vi "HitrapGUI.HTLE_TR6-UpperPart.vi"() -> ()   [LabVIEW 2014, in "HitrapGUI.lvlib"]
uses:
  HitrapGUI.lvlib
  CSlibraries/GUILib/GUILib.userEventsMainType.ctl
  CSlibraries-extern/DimLVEvent/DimIndicators/DimIndicators.anyType.ctl
  CSlibraries/GUILib/GUILib.simpleNumeric.ctl
  CSlibraries/GUILib/GUILib.basicNumeric.ctl
  CSlibraries-extern/DimLVEvent/DimIndicators/DimIndicators.numericType.ctl
  CSlibraries/UtilityLib/UtilityLib.valueStatus.ctl
  CS_Core/CSSystem/CoreDefs/CoreDefs.rawDataType.ctl
  CS_Core/CSSystem/CoreLib/CoreLib.int 2 byte array.vi
  CS_Core/CSSystem/CoreLib/CoreLib.double 2 byte array.vi
  CSlibraries/UtilityLib/UtilityLib.lvlib
  CS_Core/CSSystem/CSSystemLib/CSSystemLib.lvlib
  CSlibraries-extern/DimLVEvent/DimIndicators/DimIndicators.lvlib
  CS_Core/GUIs/GOGControllerGUI/GOGControllerGUI.lvlib
  CSlibraries/GUILib/GUILib.lvlib
  CS_Core/CSSystem/CoreLib/CoreLib.lvlib
  CSlibraries-extern/DimLVEvent/LVDimInterface/LVDimInterface.lvlib
panel:
  in  "MotorActivityLink-Act":T1
  in  "MotorLink-Act":T1
  in  "TR6DK4Link":T2
  in  "TR6DK5Link":T2
  in  "TR6ME1Ctl 2":T3 caption="TR6QME1" {"nom" step=1.0}
  in  "TR6ME1Ctl":T3 caption="TR6QME1" {"nom" step=1.0}
  in  "TR6QD4_1Ctl":T3 caption="TR6QD4_1" {"nom" step=1.0}
  in  "TR6QD4_2Ctl":T3 caption="TR6QD4_2" {"nom" step=1.0}
  in  "TR6KY5Ctl":T3 caption="TR6KY5" {"nom" step=1.0}
  in  "TR6KX5Ctl":T3 caption="TR6KX5" {"nom" step=1.0}
  in  "TR6KY4Ctl":T3 caption="TR6KY4" {"nom" step=1.0}
  in  "TR6KX4Ctl":T3 caption="TR6KX4" {"nom" step=1.0}
  in  "TR6DK5Ctl":T5 caption="TR6DK5" {"Progress Slide" scale=0.0..100.0; "Nom_Position" items=["Undefined", "Open", "Faraday Cup", "MCP"]}
  in  "TR6DK4Ctl":T5 caption="TR6DK4" {"Progress Slide" scale=0.0..100.0; "Nom_Position" items=["Undefined", "Open", "Faraday Cup", "MCP"]}
  in  "userEventsMain 2":T6
  in  "userEventsMain":T6
  in  "Next":bool
  in  "Previous":bool
  in  "analog1Ctl":T3 {"nom" step=1.0}
  in  "analog1":bool=TRUE
  out "subSystem1State":string
  in  "subSystem1":bool
  out "subSystem1StateQuality":string
  in  "subControllersIgnoredDIM":T1
  in  "iniData":string
  in  "stop":bool
  in  "dummy":bool
  in  "parentSystem":bool
  in  "userEvent":refnum<user-event>
  # "TR6-UpperPart"
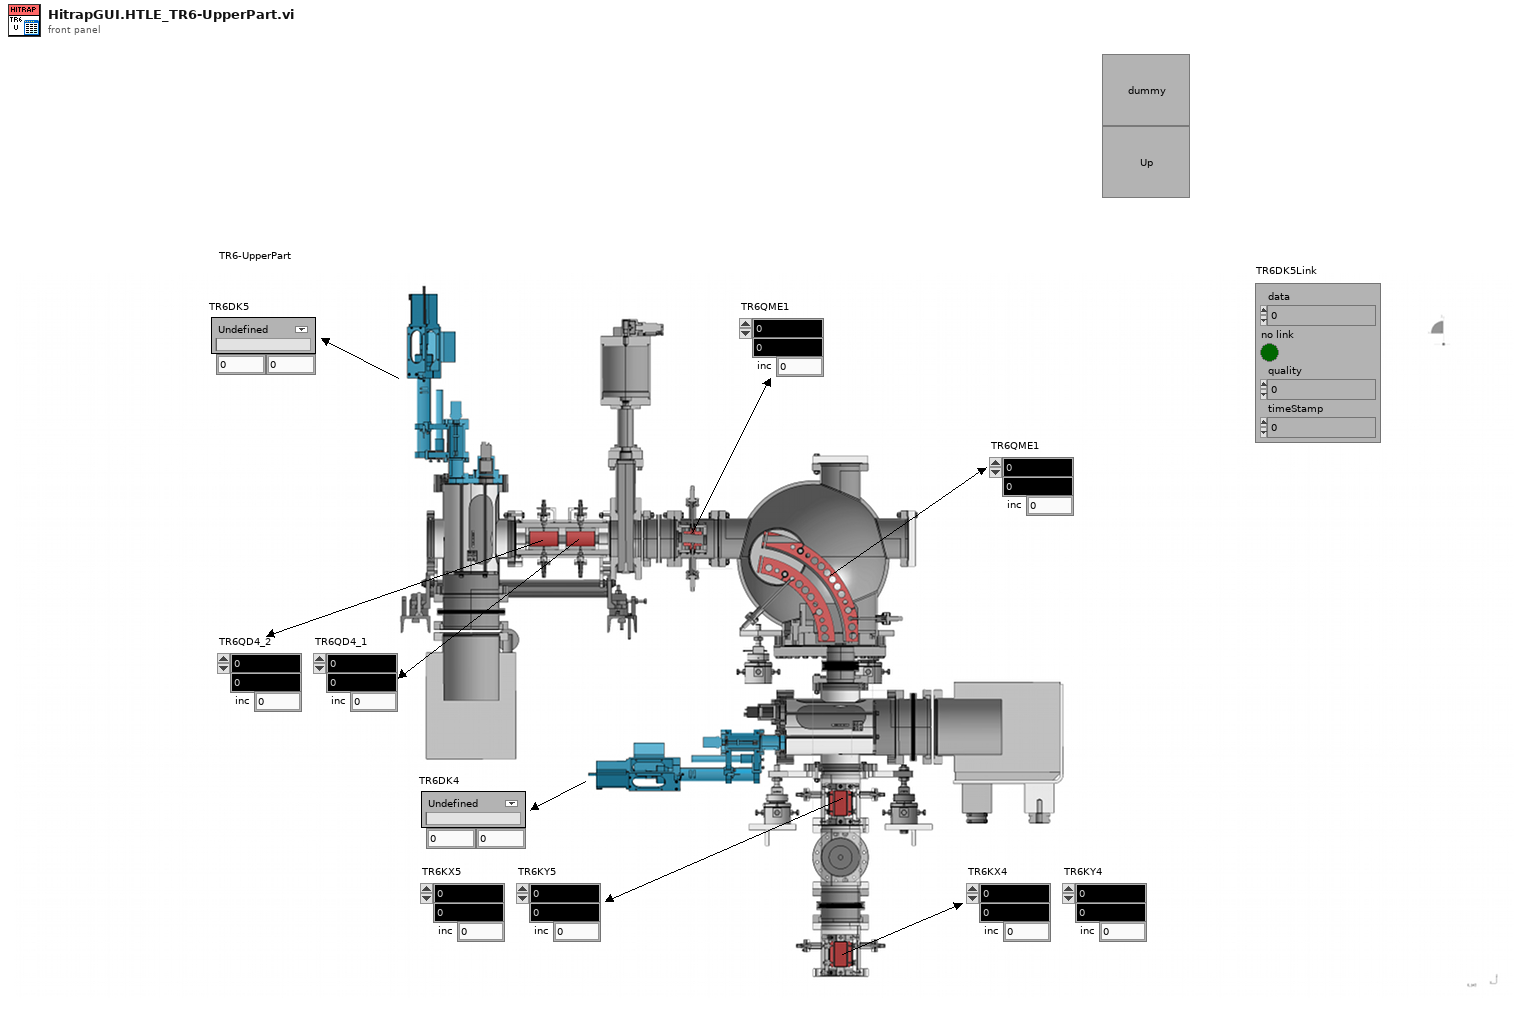
[diagram p1: front panel]
types:
  T1 = typedef "DimIndicators.lvlib/DimIndicators.anyType.ctl" = cluster{"data":string, "no link":bool, "quality":i32, "timeStamp":dbl}
  T2 = typedef "DimIndicators.lvlib/DimIndicators.numericType.ctl" = cluster{"data":dbl, "no link":bool, "quality":i32, "timeStamp":dbl}
  T3 = typedef "GUILib.lvlib/GUILib.simpleNumeric.ctl" = cluster{"nom":T4, "act":dbl, "inc":dbl}
  T4 = typedef "GUILib.lvlib/GUILib.basicNumeric.ctl" = dbl
  T5 = cluster{"Nom_Position":u8, "Progress Slide":u8, "TR6DK2Act":dbl, "TR6DK2Nom":dbl}
  T6 = typedef "GUILib.lvlib/GUILib.userEventsMainType.ctl" = cluster{"data":string, "dataType":i32}
  T7 = enum16{"Idle", "StartMotorActivity", "NewMotorDIM", "StopMotorActivity", "Stop"}
  T8 = typedef "UtilityLib.lvlib/UtilityLib.valueStatus.ctl" = enum16{"no info available", "stand by/off", "on", "warning", "alarm/malfunction", "not implemented", "user action required", "important information", "system default", "control default", "indicator default", "button default"}
  T9 = typedef "CoreDefs.rawDataType.ctl" = i8[]
  T10 = enum8{"Enabled", "Disabled", "Disabled and Grayed Out"}
  T11 = typedef "lveventtype.ctl" = enum32{"Null", "Timeout", "Annotation Menu Selection", "Annotation Menu Selection?", "App Instance Close", "App Instance Close?", "Autoscale Range Change", "Bookmark Info Change", "Cell Edit", "Cell Edit?", "Cursor Grab", "Cursor Grab?", "Cursor Menu Selection", "Cursor Menu Selection?", "Cursor Move", "Cursor Release", "Data Change", "Direction Change", "Display State Change", "Drag Ended", "Drag Enter", "Drag Leave", "Drag Over", "Drag Source Update", "Drag Starting", "Drag Starting?", "Drop", "Exec State Change", "Key Down", "Key Down?", "Key Repeat", "Key Repeat?", "Key Up", "Listbox Double Click", "Menu Activation?", "Menu Selection (App)", "Menu Selection? (App)", "Menu Selection (User)", "Mouse Down", "Mouse Down?", "Mouse Enter", "Mouse Leave", "Mouse Move", "Mouse Up", "Mouse Wheel", "NI Security User Change (App)", "Pane Size", "Panel Close", "Panel Close?", "Panel Resize", "Plot Attribute Change", "Scale Range Change", "Shortcut Menu Activation?", "Shortcut Menu Selection (App)", "Shortcut Menu Selection? (App)", "Shortcut Menu Selection (User)", "Tree Double Click", "Tree Drag", "Tree Drag?", "Tree Drop", "Tree Drop?", "Tree Item Close", "Tree Item Close?", "Tree Item Open", "Tree Item Open?", "User Event", "Value Change"}
  T12 = cluster{"TR6DK5Ctl":refnum<vi>, "byteArray out":T9}
  T13 = typedef "HitrapGUI.lvlib/HitrapGUI.i attribute.ctl" = cluster{"SVs":refnum<k21>[], "DSCIntProc":string, "MotorActivityID":i32}
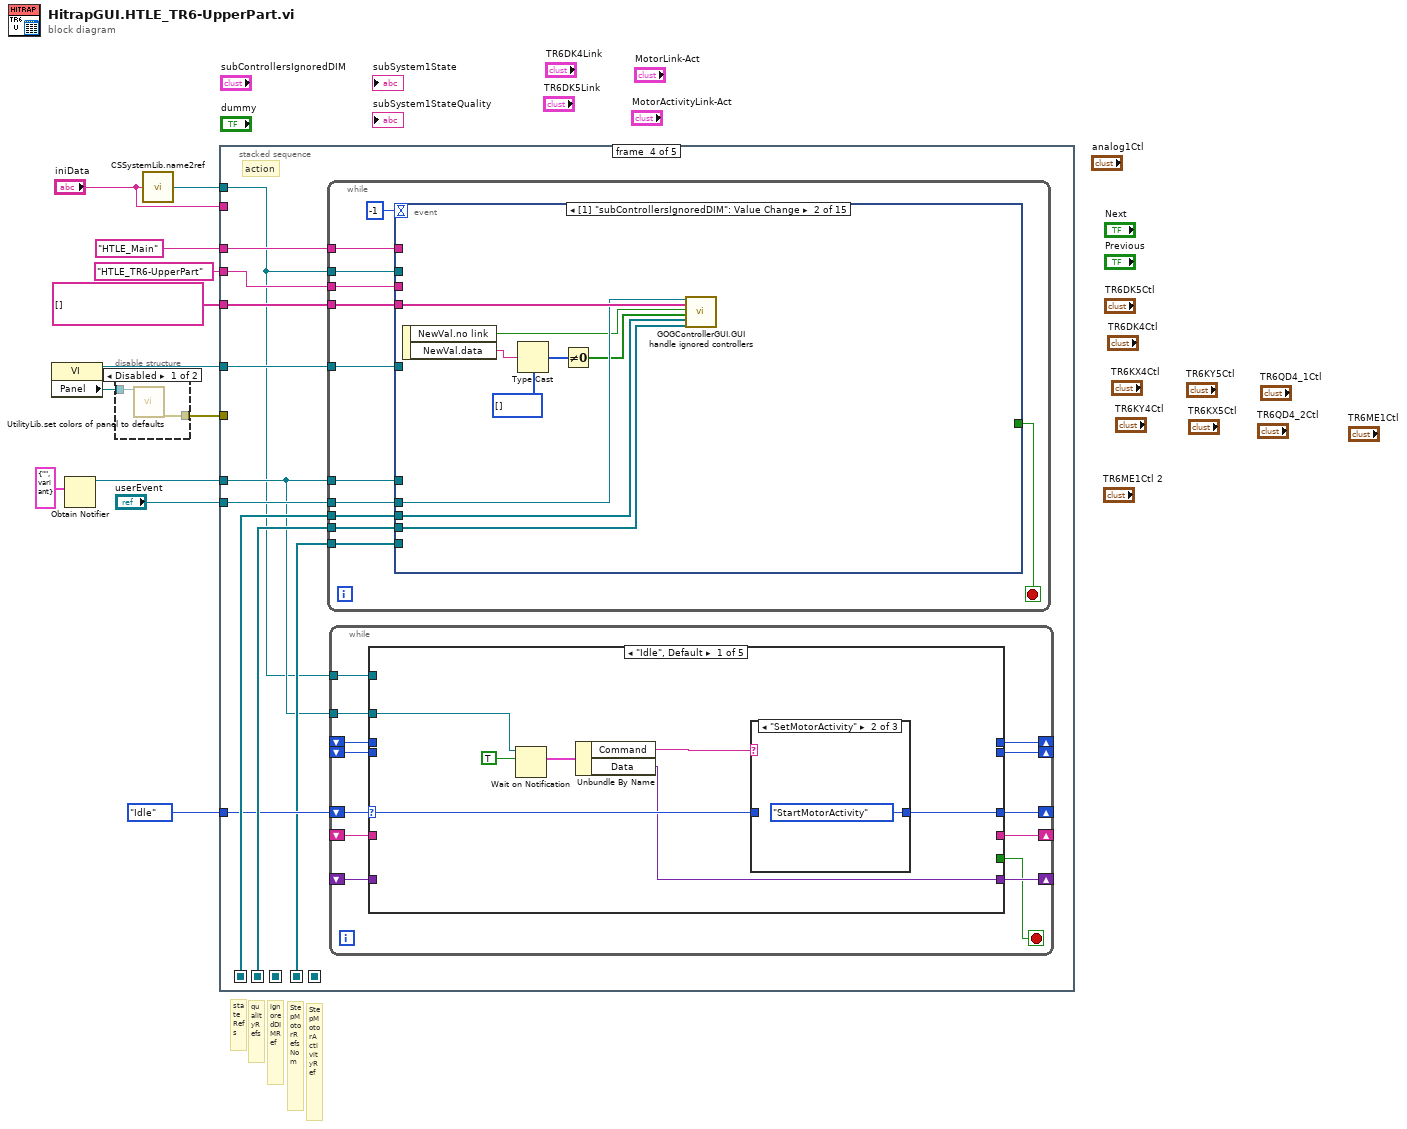
[diagram p0: block diagram]
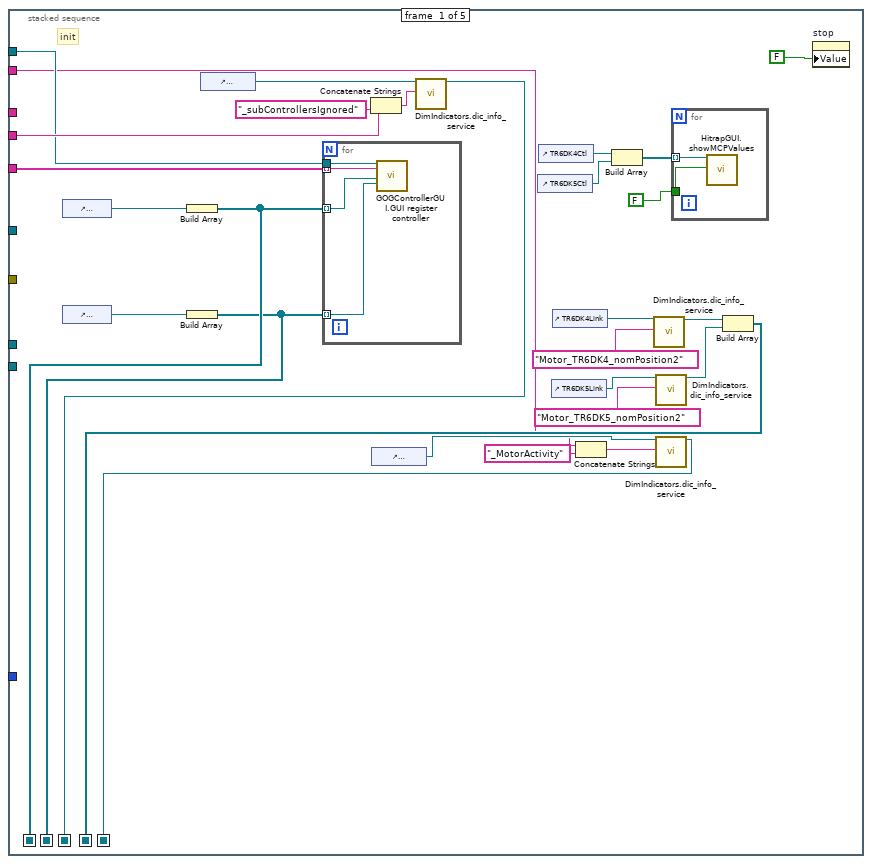
[diagram p3: hidden frame]
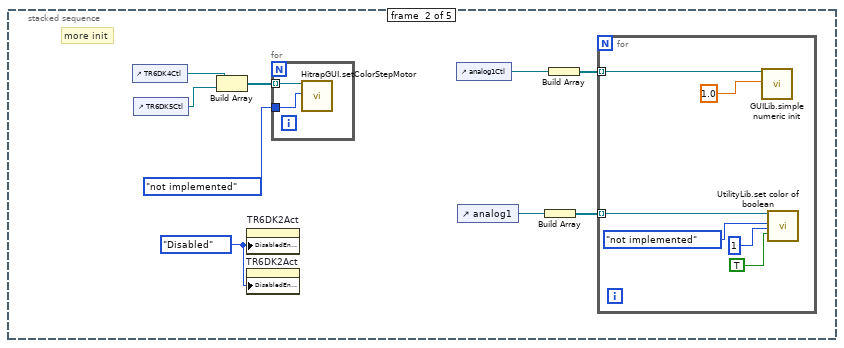
[diagram p4: hidden frame]
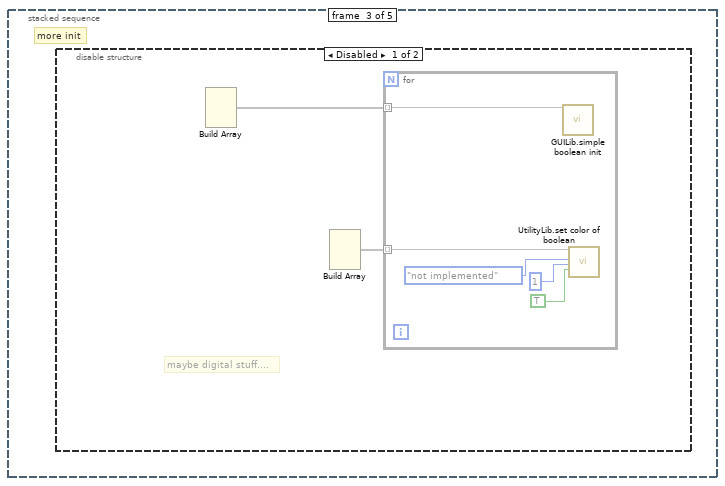
[diagram p5: hidden frame]
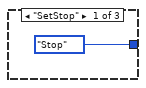
[diagram p7: hidden frame]
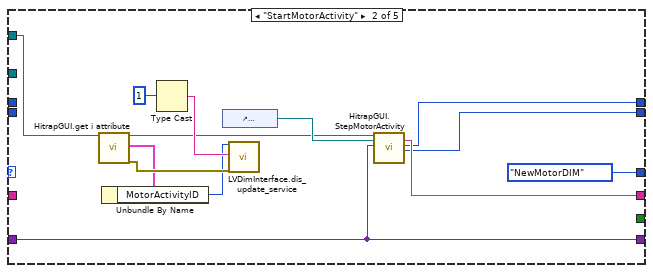
[diagram p9: hidden frame]
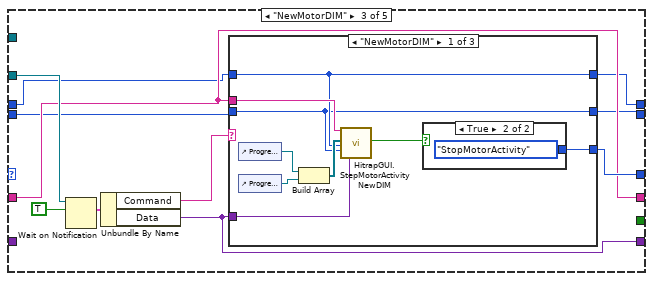
[diagram p10: hidden frame]
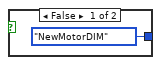
[diagram p11: hidden frame]
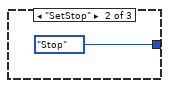
[diagram p12: hidden frame]
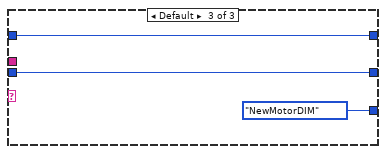
[diagram p13: hidden frame]
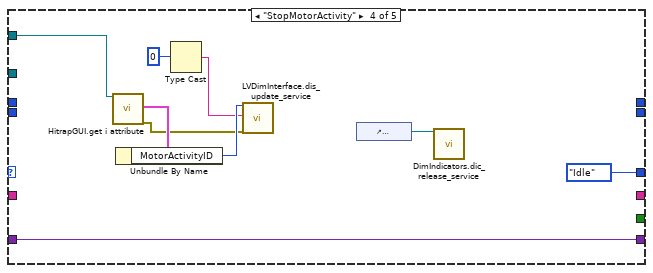
[diagram p14: hidden frame]
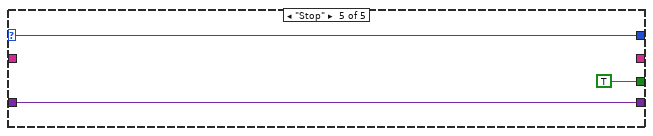
[diagram p15: hidden frame]
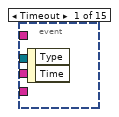
[diagram p16: hidden frame]
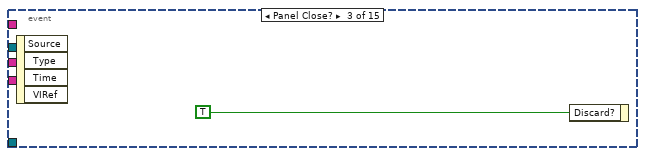
[diagram p17: hidden frame]
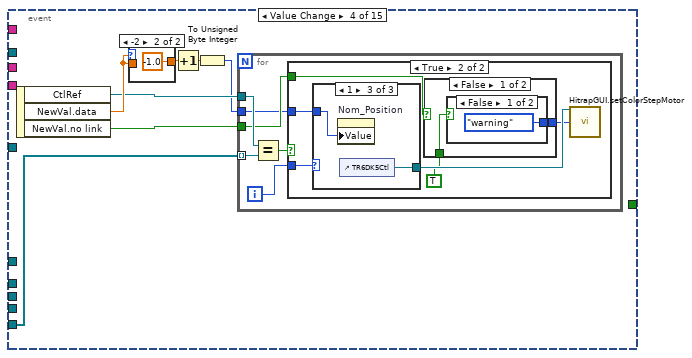
[diagram p18: hidden frame]
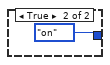
[diagram p20: hidden frame]
diagram:
  # "StepMotorActivityRef"
  # "StepMotorRefsNom"
  # "qualityRefs"
  # "ignoredDIMRef"
  # "stateRefs"
  n1 = property class="VI"() -> (reference out=w10:refnum<vi>, "Panel"=w11:refnum<vi>)  [unwired: 2 in, 1 out]
  n2 = Obtain Notifier(notification data type=cluster{"Command":string, "Data":variant} {"Command"="", "Data"=variant} ("EventData")) -> (notifier out=w1:refnum<notifier>)  [unwired: 3 in, 2 out]
  n3 = disable-structure shown="Disabled" {
    disable-tunnel: w11 -> [w14 _]
    disable-tunnel: [w13 _] -> w9
    frame Disabled {
      n4 = call "UtilityLib.set colors of panel to defaults.vi"("Front Panel"=w14) -> ("error out"=w13:errorcluster)  [unwired: 18 in]
    }
    frame Enabled {
    }
  }
  n5 = call "CSSystemLib.name2ref.vi"("name"="iniData") -> ("obj refnum"=w6:refnum<vi>)
  n6 = stacked-sequence {
    seq-local: [w32 _ _ _ _] -> [_ _ _ _ w296]
    seq-local: [w33 _ _ _ _] -> [_ _ _ w90 _]
    seq-local: [w31 _ _ _ _] -> [_ _ _ w89 _]
    seq-local: [w29 _ _ _ _] -> [_ _ _ w85 w294]
    seq-local: [w23 _ _ _ _] -> [_ _ _ _ w293]
    tunnel: "userEvent" -> [_ _ _ w93 _]
    tunnel: w10 -> [_ _ _ w92 _]
    tunnel: w9 -> [_ _ _ _ _]
    tunnel: "HTLE_TR6-UpperPart" -> [w38 _ _ w88 _]
    tunnel: string[] [] -> [w37 _ _ w91 _]
    tunnel: w6 -> [w36 _ _ w83 _]
    tunnel: "HTLE_Main" -> [_ _ _ w87 _]
    tunnel: "iniData" -> [w19 _ _ _ _]
    tunnel: T7."Idle" -> [_ _ _ w86 _]
    tunnel: w1 -> [_ _ _ w84 w295]
    frame #0 {
      # "init"
      n7 = control-ref of="dummySubSystemState"() -> (w35:refnum<vi>)
      n8 = control-ref of="dummySubSystemStateQuality"() -> (w34:refnum<vi>)
      n9 = Build Array(w35) -> (w33:refnum<vi>[])
      n10 = Build Array(w34) -> (w31:refnum<vi>[])
      n11 = control-ref of="subControllersIgnoredDIM"() -> (w39:refnum<vi>)
      n12 = for {
        tunnel: w33 -> [w48] mode=indexing
        tunnel: w37 -> [w46] mode=indexing
        tunnel: w31 -> [w45] mode=indexing
        tunnel: w36 -> [w47]
        n13 = call "GOGControllerGUI.GUI register controller.vi"("i ref in"=w47, "controllerName"=w46, "subSystemState"=w48, "subSystemStateQuality"=w45) -> ()  [unwired: 14 in, 2 out]
      }
      n14 = Concatenate Strings(w38, "_subControllersIgnored" ("string")) -> (w41:string)
      n15 = control-ref of="MotorActivityLink-Act"() -> (w20:refnum<vi>)
      n16 = call "DimIndicators.dic_info_service.vi"("controlRef"=w39, "serviceName"=w41) -> ("controlRef out"=w32:refnum<vi>)  [unwired: 16 in, 1 out]
      n17 = control-ref of="TR6DK5Ctl"() -> (w15:refnum<vi>)
      n18 = control-ref of="TR6DK4Ctl"() -> (w16:refnum<vi>)
      n19 = control-ref of="TR6DK5Link"() -> (w24:refnum<vi>)
      n20 = control-ref of="TR6DK4Link"() -> (w25:refnum<vi>)
      n21 = Concatenate Strings(w19, "_MotorActivity" ("string")) -> (w22:string)
      n22 = Build Array(w16, w15) -> (w17:refnum<vi>[])
      n23 = call "DimIndicators.dic_info_service.vi"("controlRef"=w25, "serviceName"="Motor_TR6DK4_nomPosition2") -> ("controlRef out"=w30:refnum<vi>)  [unwired: 16 in, 1 out]
      n24 = call "DimIndicators.dic_info_service.vi"("controlRef"=w24, "serviceName"="Motor_TR6DK5_nomPosition2") -> ("controlRef out"=w26:refnum<vi>)  [unwired: 16 in, 1 out]
      n25 = call "DimIndicators.dic_info_service.vi"("controlRef"=w20, "serviceName"=w22) -> ("controlRef out"=w23:refnum<vi>)  [unwired: 16 in, 1 out]
      n26 = for {
        tunnel: w17 -> [w44] mode=indexing
        tunnel: FALSE ("Visible") -> [w43]
        n27 = call "HitrapGUI.showMCPValues.vi"("Cluster Refnum"=w44, "show"=w43) -> ()  [unwired: 16 in, 2 out]
      }
      n28 = Build Array(w30, w26) -> (w29:refnum<vi>[])
      n29 = property on="stop" class="Bool (strict)"("Value"=FALSE ("stop")) -> ()  [unwired: 2 in, 2 out]
    }
    frame #1 {
      w49 = T10."Disabled" ("Disabled")
      # "more init"
      n30 = control-ref of="TR6DK4Ctl"() -> (w51:refnum<vi>)
      n31 = control-ref of="TR6DK5Ctl"() -> (w50:refnum<vi>)
      n32 = Build Array(w51, w50) -> (w52:refnum<vi>[])
      n33 = property on="TR6DK2Act" class="DigNum (strict)"("DisabledEnum"=w49) -> ()  [unwired: 2 in, 2 out]
      n34 = property on="TR6DK2Act" class="DigNum (strict)"("DisabledEnum"=w49) -> ()  [unwired: 2 in, 2 out]
      n35 = for {
        tunnel: w52 -> [w59] mode=indexing
        tunnel: UtilityLib.valueStatus."not implemented" ("State") -> [w58]
        n36 = call "HitrapGUI.setColorStepMotor.vi"("Cluster Refnum"=w59, "State"=w58) -> ()  [unwired: 16 in, 2 out]
      }
      n37 = control-ref of="analog1Ctl"() -> (w57:refnum<vi>)
      n38 = control-ref of="analog1"() -> (w55:refnum<vi>)
      n39 = Build Array(w55) -> (w54:refnum<vi>[])
      n40 = Build Array(w57) -> (w56:refnum<vi>[])
      n41 = for {
        tunnel: w56 -> [w65] mode=indexing
        tunnel: w54 -> [w61] mode=indexing
        n42 = call "GUILib.simple numeric init.vi"("ctlRef"=w65, "increment"=1.0) -> ()  [unwired: 16 in, 2 out]
        n43 = call "UtilityLib.set color of boolean.vi"("button"=w61, "valueStatus"=UtilityLib.valueStatus."not implemented", "nOfPair (0)"=1, "setTRUEColor (FALSE)"=TRUE) -> ()  [unwired: 15 in, 1 out]
      }
    }
    frame #2 {
      # "more init"
      n44 = disable-structure shown="Disabled" {
        frame Disabled {
          # "maybe digital stuff...."
          n45 = Build Array() -> (w72:void[], w77:dbl, w76:dbl, w75:dbl, w74:dbl, w73:dbl)
          n46 = Build Array() -> (w66:void[], w71:dbl, w70:dbl, w69:dbl, w68:dbl, w67:dbl)
          n47 = for {
            tunnel: w72 -> [w82] mode=indexing
            tunnel: w66 -> [w78] mode=indexing
            n48 = call "GUILib.simple boolean init.vi"("ctlRef"=w82) -> ()  [unwired: 17 in, 2 out]
            n49 = call "UtilityLib.set color of boolean.vi"("button"=w78, "valueStatus"=UtilityLib.valueStatus."not implemented", "nOfPair (0)"=1, "setTRUEColor (FALSE)"=TRUE) -> ()  [unwired: 15 in, 1 out]
          }
        }
        frame Enabled {
        }
      }
    }
    frame #3 {
      # "action"
      n50 = while {
        tunnel: w93 -> [w179]
        tunnel: w92 -> [w177]
        tunnel: w91 -> [w175]
        tunnel: w90 -> [w174]
        tunnel: w89 -> [w173]
        tunnel: w83 -> [w172]
        tunnel: w88 -> [w171]
        tunnel: w87 -> [w170]
        tunnel: w85 -> [w169]
        tunnel: w84 -> [w168]
        stop <- w176 stop-if-true
        n51 = event shown="[1] \"subControllersIgnoredDIM\": Value Change" {
          selector: _ -> [_ _ _ _ _ _ _ _ _ _ _ _ _ _ _]
          dyn-events: _ -> [_ _ _ _ _ _ _ _ _ _ _ _ _ _ _]
          timeout: -1 -> [_ _ _ _ _ _ _ _ _ _ _ _ _ _ _]
          tunnel: w179 -> [_ w184 _ _ _ _ _ _ _ w267 _ w273 w278 w283 _]
          tunnel: w177 -> [_ _ _ _ _ _ _ _ _ _ _ _ _ _ _]
          tunnel: [_ _ _ _ _ _ _ _ _ _ _ _ _ _ "stop"] -> w176
          tunnel: w175 -> [_ w185 _ _ _ _ _ _ _ w263 _ _ _ _ _]
          tunnel: w174 -> [_ w181 _ _ _ _ _ _ _ _ _ _ _ _ _]
          tunnel: w173 -> [_ w180 _ _ _ _ _ _ _ _ _ _ _ _ _]
          tunnel: w172 -> [_ _ _ _ _ _ _ _ w260 _ _ w277 _ _ _]
          tunnel: w171 -> [_ _ _ _ _ _ _ _ w258 _ _ w271 _ _ _]
          tunnel: w170 -> [_ _ _ _ _ _ _ _ _ w262 _ _ _ _ _]
          tunnel: w169 -> [_ _ _ w193 _ _ _ _ _ _ _ _ _ _ _]
          tunnel: w168 -> [_ _ _ _ _ w224 w244 _ _ _ _ _ _ _ w288]
          event Timeout {
            n52 = event-data() -> ()  [unwired: 1 in, 2 out]
          }
          event Value Change {
            n53 = event-data() -> ("NewVal.no link"=w183:bool, "NewVal.data"=w186:string)  [unwired: 1 in]
            n54 = Type Cast(type=T9 [] ("Array"), x=w186) -> (*(type *) &x=w188:T9)
            n55 = Not Equal To 0?(x=w188) -> (x != 0?=w182:bool[])
            n56 = call "GOGControllerGUI.GUI handle ignored controllers.vi"("userEvent"=w184, "controllerNames"=w185, "NOLINK"=w183, "controllersIgnored"=w182, "stateRefs"=w181, "qualityRefs"=w180) -> ()  [unwired: 14 in]
          }
          event Panel Close? {
            n57 = event-data() -> ()  [unwired: 1 in, 4 out]
            n58 = event-data("Discard?"=TRUE) -> ()  [unwired: 1 in, 1 out]
          }
          event Value Change {
            n59 = event-data() -> ("CtlRef"=w191:refnum<vi>, "NewVal.data"=w194:dbl, "NewVal.no link"=w192:bool)  [unwired: 1 in]
            n60 = case shown="-2" w194 {
              tunnel: [w218 -1.0] -> w196
              tunnel: w194 -> [w218 _]
              frame 0, Default {
              }
              frame -2 {
              }
            }
            n61 = Increment(x=w196) -> (x+1=w195:dbl)
            n62 = To Unsigned Byte Integer(number=w195) -> (unsigned 8bit integer=w190:u8)
            n63 = for {
              tunnel: w193 -> [w202] mode=indexing
              tunnel: w192 -> [w198]
              tunnel: w191 -> [w201]
              tunnel: w190 -> [w197]
              i -> [w199]
              n64 = Equal?(x=w201, y=w202) -> (x = y?=w200:bool)
              n65 = case shown="True" w200 {
                tunnel: w199 -> [_ w208]
                tunnel: w198 -> [_ w207]
                tunnel: w197 -> [_ w206]
                frame False {
                }
                frame True {
                  n66 = case shown="1" w208 {
                    tunnel: w206 -> [_ w215 w216]
                    tunnel: [_ w214 w217] -> w205
                    frame Default {
                    }
                    frame 0 {
                      n67 = property on="Nom_Position" class="Ring (strict)"("Value"=w215) -> ()  [unwired: 2 in, 2 out]
                      n68 = control-ref of="TR6DK4Ctl"() -> (w214:refnum<vi>)
                    }
                    frame 1 {
                      n69 = property on="Nom_Position" class="Ring (strict)"("Value"=w216) -> ()  [unwired: 2 in, 2 out]
                      n70 = control-ref of="TR6DK5Ctl"() -> (w217:refnum<vi>)
                    }
                  }
                  n71 = case shown="False" w207 {
                    tunnel: [w210 UtilityLib.valueStatus."not implemented" ("State")] -> w204
                    tunnel: TRUE -> [w209 _]
                    frame False {
                      n72 = case shown="False" w209 {
                        tunnel: [UtilityLib.valueStatus."warning" ("State") UtilityLib.valueStatus."on" ("State")] -> w210
                        frame False {
                        }
                        frame True {
                        }
                      }
                    }
                    frame True {
                    }
                  }
                  n73 = call "HitrapGUI.setColorStepMotor.vi"("Cluster Refnum"=w205, "State"=w204) -> ()  [unwired: 16 in, 2 out]
                }
              }
            }
          }
          event "TR6DK4Ctl", "TR6DK5Ctl": Mouse Enter; "TR6DK4Ctl", "TR6DK5Ctl": Mouse Leave {
            n74 = event-data() -> ("CtlRef"=w220:refnum<vi>, "Type"=w221:T11)  [unwired: 1 in]
            n75 = case shown="\"Mouse Enter\"" w221 {
              tunnel: [TRUE _] -> w222
              frame "Mouse Enter" {
              }
              frame Default {
              }
            }
            n76 = call "HitrapGUI.showMCPValues.vi"("Cluster Refnum"=w220, "show"=w222) -> ()  [unwired: 16 in, 2 out]
          }
          event "TR6DK4Ctl.Nom_Position", "TR6DK5Ctl.Nom_Position": Value Change {
            n77 = event-data() -> ("CtlRef"=w227:refnum<vi>, "NewVal"=w226:u8)  [unwired: 1 in, 1 out]
            n78 = Greater Than 0?(x=w226) -> (x > 0?=w225:bool)
            n79 = case shown="True" w225 {
              tunnel: w227 -> [_ w240]
              tunnel: w226 -> [_ w241]
              tunnel: w224 -> [_ w239]
              frame False {
              }
              frame True {
                n80 = Decrement(x=w241) -> (x-1=w232:u8)
                n81 = property class="Ring (strict)"(reference=w240) -> ("Owner"=w230:refnum<vi>)  [unwired: 1 in, 2 out]
                n82 = call-poly "CoreLib.data 2 byte array.vi"("i32"=0) -> ("byteArray out"=w234:T9)  [unwired: 18 in]
                n83 = call-poly "CoreLib.data 2 byte array.vi"("byteArray"=w234, "i32"=w232) -> ("byteArray out"=w231:T9)  [unwired: 17 in]
                n84 = control-ref of="TR6DK5Ctl"() -> (w228:refnum<vi>)
                n85 = To More Specific Class(target class=w228, reference=w230) -> (specific class reference=w229:refnum<vi>)  [unwired: 1 in, 1 out]
                n86 = Bundle("TR6DK5Ctl"=w229, "byteArray out"=w231) -> (w235:T12)  [unwired: 1 in]
                n87 = To Variant(anything=w235) -> (Variant=w236:variant)
                n88 = Bundle("SetMotorActivity", "Variant"=w236) -> (w238:cluster{string, "Variant":variant})  [unwired: 1 in]
                n89 = Send Notification(notification=w238, notifier=w239) -> ()  [unwired: 1 in, 2 out]
              }
            }
          }
          event Value Change {
            w246 = 0.0
            n90 = event-data() -> ("OldVal"=w242:string, "NewVal"=w243:string)  [unwired: 1 in, 1 out]
            n91 = Type Cast(type=w246, x=w243) -> (*(type *) &x=w245:dbl)
            n92 = Type Cast(type=w246, x=w242) -> (*(type *) &x=w247:dbl)
            n93 = Bundle(w247, w245) -> (w248:cluster{dbl, dbl})  [unwired: 1 in]
            n94 = To Variant(anything=w248) -> (Variant=w249:variant)
            n95 = Bundle("NewMotorDIM", "Variant"=w249) -> (w251:cluster{string, "Variant":variant})  [unwired: 1 in]
            n96 = Send Notification(notification=w251, notifier=w244) -> ()  [unwired: 1 in, 2 out]
          }
          event Value Change {
            n97 = event-data() -> ("NewVal"=w253:string)  [unwired: 1 in, 2 out]
            n98 = Type Cast(type=i16 0 ("x"), x=w253) -> (*(type *) &x=w254:i16)
            n99 = case shown="0, Default" w254 {
              tunnel: [T10."Enabled" ("Disabled") T10."Disabled and Grayed Out" ("Disabled")] -> w252
              frame 0, Default {
              }
              frame 1 {
              }
            }
            n100 = property on="TR6DK5Ctl" class="Clust (strict)"("DisabledEnum"=w252) -> ()  [unwired: 2 in, 2 out]
            n101 = property on="TR6DK4Ctl" class="Clust (strict)"("DisabledEnum"=w252) -> ()  [unwired: 2 in, 2 out]
          }
          event "analog1": Value Change {
            n102 = event-data() -> ("CtlRef"=w259:refnum<vi>)  [unwired: 1 in]
            n103 = call "GOGControllerGUI.GUI open front panel.vi"("i ref in"=w260, "elementRef"=w259, "controller"=w258) -> ()  [unwired: 15 in, 2 out]
          }
          event "subSystem1", "parentSystem": Value Change {
            n104 = event-data() -> ("CtlRef"=w265:refnum<vi>)  [unwired: 1 in]
            n105 = control-ref of="parentSystem"() -> (w264:refnum<vi>)
            n106 = control-ref of="subSystem1"() -> (w268:refnum<vi>)
            n107 = Build Array (concatenate)(w262, w263) -> (w261:string[])
            n108 = Build Array(w264, w268) -> (w266:refnum<vi>[])
            n109 = call "GOGControllerGUI.GUI set selected subcontroller.vi"("userEvent"=w267, "controllerNames"=w261, "controllerRefs"=w266, "controllerRef"=w265) -> ()  [unwired: 16 in]
          }
          event Value Change {
            n110 = event-data() -> ("CtlRef"=w270:refnum<vi>, "NewVal"=w269:dbl)  [unwired: 1 in]
            n111 = call "GUILib.simple numeric change increment.vi"("ctlRef"=w270, "increment"=w269) -> ()  [unwired: 16 in, 2 out]
          }
          event Value Change {
            n112 = event-data() -> ("CtlRef"=w276:refnum<vi>, "NewVal"=w275:T4)  [unwired: 1 in]
            n113 = call-poly "CoreLib.data 2 byte array.vi"("f64"=w275) -> ("byteArray out"=w274:T9)  [unwired: 18 in]
            n114 = call "GOGControllerGUI.GUI set nominal value.vi"("i ref in"=w277, "nominalRef"=w276, "nominalData"=w274, "controller"=w271) -> ("error out"=w272:errorcluster)  [unwired: 14 in, 1 out]
            n115 = call "GOGControllerGUI.GUI set error.vi"("userEvent"=w273, "controller"=w271, "GUIError"=w272) -> ()  [unwired: 16 in, 1 out]
          }
          event "Previous": Value Change {
            n116 = event-data() -> ()  [unwired: 1 in, 3 out]
            n117 = Bundle By Name(cluster="userEventsMain", "data"="HTLE_TR6-LowerPart", "dataType"=0) -> (w282:T6)
            n118 = Generate User Event(user event=w278, event data cluster=w282) -> ()  [unwired: 2 in, 2 out]
          }
          event "Next": Value Change {
            n119 = event-data() -> ()  [unwired: 1 in, 3 out]
            n120 = Bundle By Name(cluster="userEventsMain 2", "data"="HTLE_TR7", "dataType"=0) -> (w287:T6)
            n121 = Generate User Event(user event=w283, event data cluster=w287) -> ()  [unwired: 2 in, 2 out]
          }
          event "stop": Value Change {
            n122 = event-data() -> ()  [unwired: 1 in, 6 out]
            n123 = Bundle("SetStop", "Data"=variant) -> (w291:cluster{string, "Data":variant})  [unwired: 1 in]
            n124 = Send Notification(notification=w291, notifier=w288) -> ()  [unwired: 1 in, 2 out]
          }
        }
      }
      n125 = while {
        shift-right: [w104] -> _
        shift-left: w86 -> [w106]
        tunnel: w84 -> [w105]
        shift-right: [w103] -> _
        shift-left: _ -> [w101]
        tunnel: w83 -> [w102]
        shift-right: [w100] -> _
        shift-left: _ -> [w94]
        shift-right: [w99] -> _
        shift-left: _ -> [w96]
        shift-right: [w98] -> _
        shift-left: _ -> [w95]
        stop <- w97 stop-if-true
        n126 = case shown="\"Idle\", Default" w106 {
          selector: w106 -> [w110 _ _ _ w167]
          tunnel: w105 -> [w107 _ w137 _ _]
          tunnel: [w109 T7."NewMotorDIM" w136 T7."Idle" w167] -> w104
          tunnel: [w108 w121 w135 w156 w166] -> w103
          tunnel: w102 -> [_ w122 _ w157 _]
          tunnel: w101 -> [_ w121 _ w156 w166]
          tunnel: [_ w119 w134 _ _] -> w100
          tunnel: [_ w118 w131 _ _] -> w99
          tunnel: [_ w117 w130 _ _] -> w98
          tunnel: [_ _ _ _ TRUE] -> w97
          tunnel: w96 -> [_ _ w133 _ _]
          tunnel: w95 -> [_ _ w132 _ _]
          tunnel: w94 -> [_ _ w134 _ _]
          frame "Idle", Default {
            n127 = Wait on Notification(notifier=w107, ignore previous (F)=TRUE) -> (notification=w113:cluster{"Command":string, "Data":variant})  [unwired: 2 in, 3 out]
            n128 = Unbundle By Name(w113) -> ("Command"=w112:string, "Data"=w108:variant)
            n129 = case shown="\"SetMotorActivity\"" w112 {
              tunnel: w110 -> [_ _ w116]
              tunnel: [T7."Stop" T7."StartMotorActivity" w116] -> w109
              frame "SetStop" {
              }
              frame "SetMotorActivity" {
              }
              frame "Idle", Default {
              }
            }
          }
          frame "StartMotorActivity" {
            n130 = call "HitrapGUI.get i attribute.vi"("i ref in"=w122) -> ("i ref out"=w123:refnum<vi>, "i attribute"=w124:T13, "error out"=w126:errorcluster)  [unwired: 16 in]
            n131 = Unbundle By Name(w124) -> ("MotorActivityID"=w125:i32)
            n132 = Type Cast(x=i16 1) -> (*(type *) &x=w128:string)  [unwired: 1 in]
            n133 = control-ref of="MotorLink-Act"() -> (w129:refnum<vi>)
            n134 = call "LVDimInterface.dis_update_service.vi"("my_serviceID"=w125, "data"=w128, "error in (no error)"=w126) -> ()  [unwired: 14 in, 3 out]
            n135 = call "HitrapGUI.StepMotorActivity.vi"("i ref in"=w123, "DIMPositioncontrolRef"=w129, "Data"=w121) -> ("MotorName"=w119:string, "StartPosition"=w118:i32, "StopPosition"=w117:i32)  [unwired: 12 in, 2 out]
          }
          frame "NewMotorDIM" {
            n136 = Wait on Notification(notifier=w137, ignore previous (F)=TRUE) -> (notification=w139:cluster{"Command":string, "Data":variant})  [unwired: 2 in, 3 out]
            n137 = Unbundle By Name(w139) -> ("Command"=w140:string, "Data"=w135:variant)
            n138 = case shown="\"NewMotorDIM\"" w140 {
              tunnel: [w149 T7."Stop" T7."NewMotorDIM"] -> w136
              tunnel: w133 -> [w144 _ w154]
              tunnel: w132 -> [w143 _ w153]
              tunnel: w135 -> [w146 _ _]
              tunnel: w134 -> [w145 _ _]
              tunnel: [w144 _ w154] -> w131
              tunnel: [w143 _ w153] -> w130
              frame "NewMotorDIM" {
                n139 = control-ref of="Progress Slide"() -> (w141:refnum<vi>)
                n140 = control-ref of="Progress Slide"() -> (w142:refnum<vi>)
                n141 = Build Array(w141, w142) -> (w147:refnum<vi>[])
                n142 = call "HitrapGUI.StepMotorActivityNewDIM.vi"("MotorName"=w145, "Progress Slide Array"=w147, "StartPosition"=w144, "StopPosition"=w143, "Data"=w146) -> ("Finished?"=w148:bool)  [unwired: 12 in, 2 out]
                n143 = case shown="True" w148 {
                  tunnel: [T7."NewMotorDIM" T7."StopMotorActivity"] -> w149
                  frame False {
                  }
                  frame True {
                  }
                }
              }
              frame "SetStop" {
              }
              frame Default {
              }
            }
          }
          frame "StopMotorActivity" {
            n144 = call "HitrapGUI.get i attribute.vi"("i ref in"=w157) -> ("i attribute"=w162:T13, "error out"=w160:errorcluster)  [unwired: 16 in, 1 out]
            n145 = Unbundle By Name(w162) -> ("MotorActivityID"=w161:i32)
            n146 = Type Cast(x=i16 0) -> (*(type *) &x=w158:string)  [unwired: 1 in]
            n147 = call "LVDimInterface.dis_update_service.vi"("my_serviceID"=w161, "data"=w158, "error in (no error)"=w160) -> ()  [unwired: 14 in, 3 out]
            n148 = control-ref of="MotorLink-Act"() -> (w163:refnum<vi>)
            n149 = call "DimIndicators.dic_release_service.vi"("controlRef"=w163) -> ()  [unwired: 18 in, 1 out]
          }
          frame "Stop" {
          }
        }
      }
    }
    frame #4 {
      # "deinit"
      n150 = Release Notifier(notifier=w295) -> ()  [unwired: 2 in, 3 out]
      n151 = for {
        tunnel: w294 -> [w297] mode=indexing
        n152 = call "DimIndicators.dic_release_service.vi"("controlRef"=w297) -> ()  [unwired: 18 in, 1 out]
      }
      n153 = call "DimIndicators.dic_release_service.vi"("controlRef"=w296) -> ()  [unwired: 18 in, 1 out]
      n154 = call "DimIndicators.dic_release_service.vi"("controlRef"=w293) -> ()  [unwired: 18 in, 1 out]
    }
  }
